vi "RightArmPosition.vi"(0 "error in":errorcluster, 2 "Arm Angles (degrees)":T1, 3 "node":string) -> (1 "error out":errorcluster)   [LabVIEW 2012]
doc: "Move Baxter's arm to given joint positions"
uses:
  <userlib>/ROS for LabVIEW Software/ROS/Code/SubVIs/BaxterArmsSmall.ctl
  <userlib>/ROS for LabVIEW Software/ROS/Code/SubVIs/JointMode.ctl
  <userlib>/ROS for LabVIEW Software/ROS/Code/SubVIs/BaxterSide.ctl
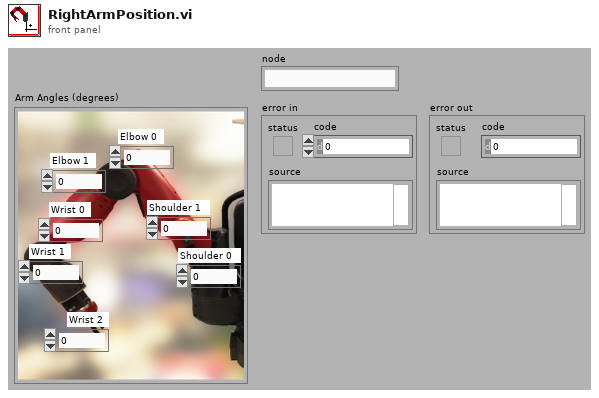
[diagram p1: front panel]
types:
  T1 = typedef "BaxterArmsSmall.ctl" = cluster{"Elbow 0":dbl, "Elbow 1":dbl, "Shoulder 0":dbl, "Shoulder 1":dbl, "Wrist 0":dbl, "Wrist 1":dbl, "Wrist 2":dbl}
  T2 = typedef "BaxterSide.ctl" = enum16{"left", "right"}
  T3 = typedef "JointMode.ctl" = u8
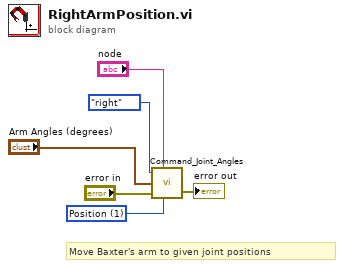
[diagram p0: block diagram]
diagram:
  w2 = T3 1 items=["Position"=1, "Velocity"=2, "Effort"=3] ("Mode")
  # "Move Baxter's arm to given joint positions"
  n1 = call <userlib>:"Command_Joint_Angles.vi"("Side"=BaxterSide."right", "node"="node", "Arm Angles (degrees)"="Arm Angles (degrees)", "error in"="error in", "Mode"=w2) -> ("error out"=→"error out":errorcluster)  [unwired: 1 in]
